vi "Fetch Measurement (Delta Time).vi"(0 "VISA resource name":refnum<visa-resource-name>, 5 "Measurement Source 1 (1: Channel 1)":i32(ring)=1 caption="Channel (1: Channel 1)" items=["Channel 1"=1, "Channel 2"=2, "Channel 3"=3, "Channel 4"=4, "Function 1"=5, "Function 2"=6, "Function 3"=7, "Function 4"=8, "Memory 1"=9, "Memory 2"=10, "Memory 3"=11, "Memory 4"=12, "Clock"=15, "MTrend"=16, "MSpectrum"=17, "Equalized"=18, "DIG 0"=20, "DIG 1"=21, "DIG 2"=22, "DIG 3"=23, "DIG 4"=24, "DIG 5"=25, "DIG 6"=26, "DIG 7"=27, "DIG 8"=28, "DIG 9"=29, "DIG 10"=30, "DIG 11"=31, "DIG 12"=32, "DIG 13"=33, "DIG 14"=34, "DIG 15"=35], 7 "Measurement Source 2 (2: Channel 2)":i32(ring)=2 caption="Channel (1: Channel 1)" items=["Channel 1"=1, "Channel 2"=2, "Channel 3"=3, "Channel 4"=4, "Function 1"=5, "Function 2"=6, "Function 3"=7, "Function 4"=8, "Memory 1"=9, "Memory 2"=10, "Memory 3"=11, "Memory 4"=12, "Clock"=15, "MTrend"=16, "MSpectrum"=17, "Equalized"=18, "DIG 0"=20, "DIG 1"=21, "DIG 2"=22, "DIG 3"=23, "DIG 4"=24, "DIG 5"=25, "DIG 6"=26, "DIG 7"=27, "DIG 8"=28, "DIG 9"=29, "DIG 10"=30, "DIG 11"=31, "DIG 12"=32, "DIG 13"=33, "DIG 14"=34, "DIG 15"=35], 11 "error in (no error)":errorcluster) -> (4 "VISA resource name out":refnum<visa-resource-name>, 6 "Delta Time(s)":dbl, 15 "error out":errorcluster)   [LabVIEW 2020, in "Agilent 90000 Series.lvlib"]
doc: "Obtains a waveform measurement (delta time between two edges) and returns the measurement value. The waveform on which the oscilloscope calculates the waveform measurement is from an acquisition that you previously initiated. \n\nUse the Initiate Acquisition VI to start an acquisition on the channels that you enable with the Configure Channel VI. The oscilloscope acquires waveforms for the enabled channels concurrently. You use the Wait For Operation Complete VI to wait for operation complete. You call this VI separately for each waveform measurement you want to obtain on a specific channel.\n\nYou can call the Read Measurement VI instead of the Initiate Acquisition VI. The Read Measurement VI starts an acquisition on all enabled channels. It then waits for the acquisition to complete, obtains a waveform measurement on the channel you specify, and returns the measurement value. You call this VI separately for any other waveform measurement that you want to obtain on a specific channel.\n\nNotes:\n\n(1) You must configure the appropriate reference levels before you call this VI to take measurement.\n\n(2) You configure the low, mid, and high references either by calling the Configure Reference Levels VI.\n\n\n(3) This VI does not check the instrument status. Typically, you call this VI only in a sequence of calls to other low-level driver VIs. The sequence performs one operation. You use the low-level VIs to optimize one or more aspects of interaction with the instrument. If you want to check the instrument status, call the Error-Query VI at the conclusion of the sequence."
uses:
  Agilent 90000 Series.lvlib
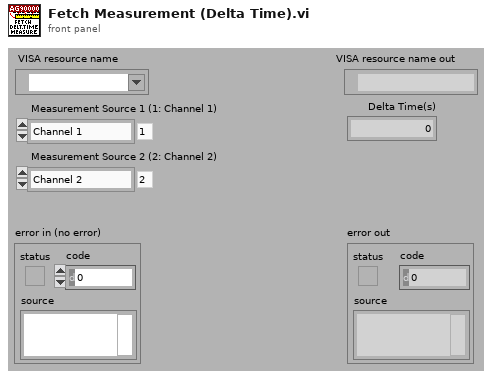
[diagram p1: front panel]
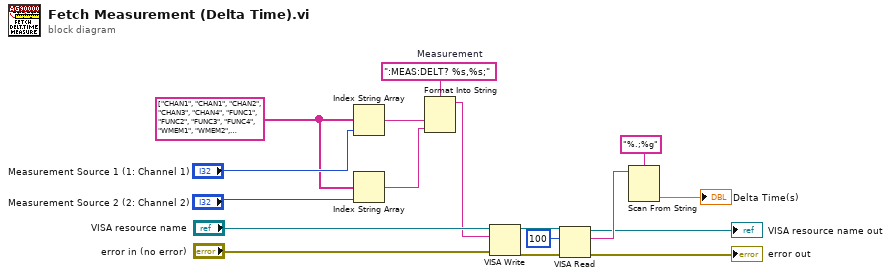
[diagram p0: block diagram]
diagram:
  w1 = string[] ["CHAN1", "CHAN1", "CHAN2", "CHAN3", "CHAN4", "FUNC1", "FUNC2", "FUNC3", "FUNC4", "WMEM1", "WMEM2", "WMEM3", "WMEM4", "AUX", "LINE", "CLOC", "MTR", "MSP", "EQU", "NONE", "DIG0", "DIG1", "DIG2", "DIG3", "DIG4", "DIG5", "DIG6", "DIG7", "DIG8", "DIG9", "DIG10", "DIG11", "DIG12", "DIG13", "DIG14", "DIG15", "", "", "", "", "", "POD1", "POD2", "", "", "", "", "", "", "", "", "BUS1", "BUS2", "BUS3", "BUS4", "", "", "", "", "", "", "DIFF1", "DIFF2", "", "", "", "", "", "", "", "", "COMM3", "COMM4"]
  w17 = ":MEAS:DELT? %s,%s;"  # Measurement
  n1 = Index String Array(1:"Measurement Source 1 (1: Channel 1)", 2:w1) -> (0:w16:string)  [unwired: 1 out]
  n2 = Index String Array(1:"Measurement Source 2 (2: Channel 2)", 2:w1) -> (0:w15:string)  [unwired: 1 out]
  n3 = Format Into String(format string=w17, w16, w15) -> (resulting string=w5:string)  [unwired: 2 in, 1 out]
  n4 = VISA Write(VISA resource name="VISA resource name", write buffer=w5, error in (no error)="error in (no error)") -> (VISA resource name out=w10:refnum<visa-resource-name>, error out=w11:errorcluster)  [unwired: 1 out]
  n5 = VISA Read(VISA resource name=w10, byte count=u32 100, error in (no error)=w11) -> (VISA resource name out=→"VISA resource name out":refnum<visa-resource-name>, read buffer=w13:string, error out=→"error out":errorcluster)  [unwired: 1 out]
  n6 = Scan From String(format string="%.;%g", input string=w13) -> (output 1=→"Delta Time(s)":dbl)  [unwired: 2 in, 4 out]
